vi "excel_creacion_archivo.vi"(7 "número":string="0", 8 "error in (no error)":errorcluster, 9 "inicial archivo":string="test_", 10 "direccion carpeta":path=path "C:/Excel", 11 "títulos columnas":string) -> (0 "error out":errorcluster, 3 "Referencia Excel":refnum<file>)   [LabVIEW 2026]
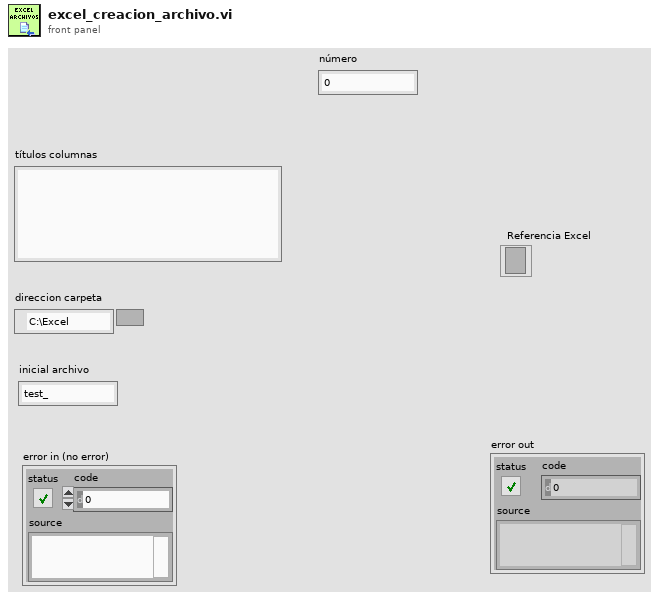
[diagram p1: front panel]
types:
  T1 = enum16{"open", "replace", "create", "open or create", "replace or create", "replace or create with confirmation"}
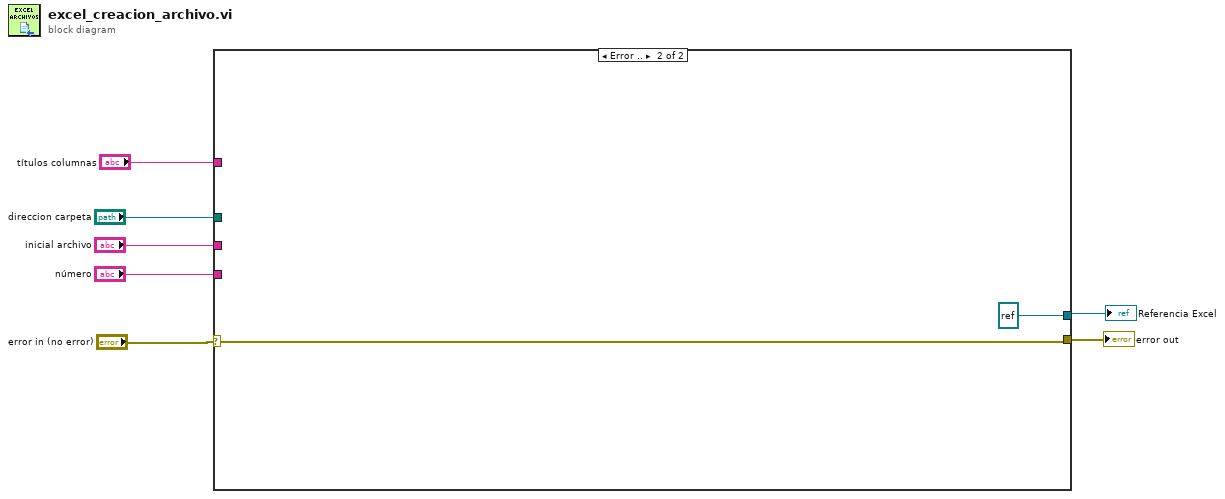
[diagram p0: block diagram]
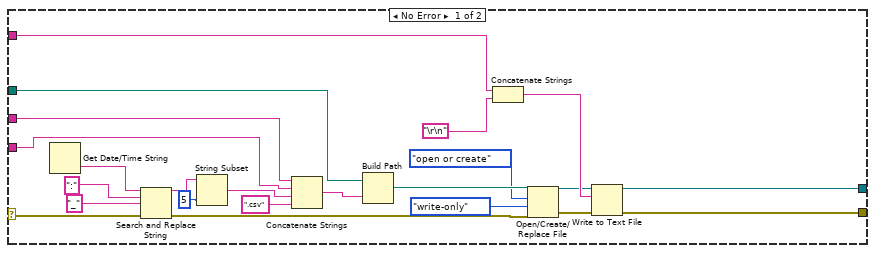
[diagram p2: hidden frame]
diagram:
  n1 = case shown="Error .." "error in (no error)" {
    selector: "error in (no error)" -> [w12 w32]
    tunnel: [w25 refnum<file> refnum ("refnum out")] -> w7
    tunnel: [w24 w32] -> w6
    tunnel: "inicial archivo" -> [w10 _]
    tunnel: "direccion carpeta" -> [w8 _]
    tunnel: "títulos columnas" -> [w11 _]
    tunnel: "número" -> [w9 _]
    frame No Error {
      n2 = Get Date/Time String() -> (time string=w15:string)  [unwired: 3 in, 1 out]
      n3 = Search and Replace String(input string=w15, search string=":", replace string="_" ("replace string (\"\")"), error in=w12) -> (result string=w28:string, error out=w20:errorcluster)  [unwired: 4 in, 2 out]
      n4 = String Subset(string=w28, length (rest)=5 ("length (rest)")) -> (substring=w30:string)  [unwired: 1 in]
      n5 = Concatenate Strings(w10, w9, w30, ".csv" ("string")) -> (w19:string)
      n6 = Build Path(base path=w8, name or relative path=w19) -> (appended path=w21:path)
      n7 = Concatenate Strings(w11, "\r\n") -> (w27:string)
      n8 = Open/Create/Replace File(file path (use dialog)=w21, error in=w20, operation (0:open)=T1."open or create", access (0:read/write)=enum16{"read/write", "read-only", "write-only"}."write-only") -> (refnum out=w22:refnum<file>, error out=w23:errorcluster)  [unwired: 2 in, 1 out]
      n9 = Write to Text File(file (use dialog)=w22, text=w27, error in=w23) -> (refnum out=w25:refnum<file>, error out=w24:errorcluster)  [unwired: 1 in, 1 out]
    }
    frame Error {
    }
  }
  "Referencia Excel" <- w7
  "error out" <- w6
